vi "HexToDate.vi"(11 "数组":u16[](array[numeric]) format="%04xH") -> (3 "DATE":timestamp[](array[timestamp]))   [LabVIEW 2016, in "斯坦道总磷.lvlib"]
uses:
  <vilib>/Utility/miscctls.llb/LVDateTimeRec.ctl
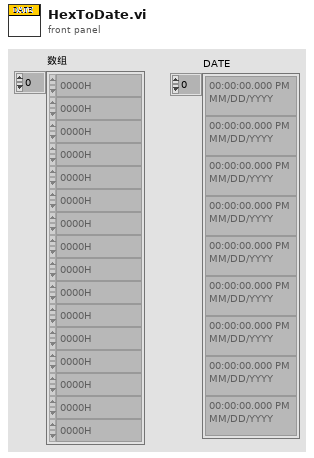
[diagram p1: front panel]
types:
  T1 = typedef "LVDateTimeRec.ctl" = cluster{"fractional second":dbl, "second":i32, "minute":i32, "hour":i32, "day of month":i32, "month":i32, "year":i32, "day of week":i32, "day of year":i32, "DST":i32}
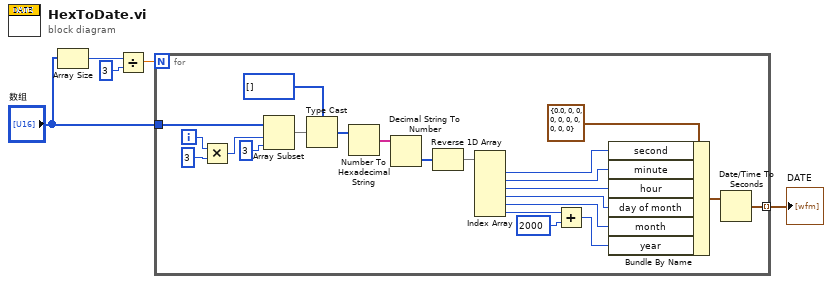
[diagram p0: block diagram]
diagram:
  n1 = Array Size(array="数组") -> (size(s)=w5:i32)
  n2 = Divide(x=w5, y=3) -> (x/y=w3:dbl)
  n3 = for {
    N: w3 -> [_]
    tunnel: "数组" -> [w27]
    tunnel: [w10] -> w1 mode=indexing
    i -> [w26]
    n4 = Multiply(x=w26, y=3) -> (x*y=w23:i32)
    n5 = Array Subset(array=w27, index=w23, length=3 ("索引")) -> (w22:u16[])
    n6 = Type Cast(type=u8[] [], x=w22) -> (*(type *) &x=w8:u8[])
    n7 = Number To Hexadecimal String(2:w8) -> (0:w7:string[])  [unwired: 1 in]
    n8 = Decimal String To Number(string=w7) -> (number=w6:i32[])  [unwired: 2 in, 1 out]
    n9 = Reverse 1D Array(array=w6) -> (reversed array=w9:i32[])
    n10 = Index Array(array=w9) -> (element #1=w19:i32, element #2=w18:i32, element #3=w17:i32, element #4=w16:i32, element #5=w15:i32, element #6=w14:i32)  [unwired: 6 in]
    n11 = Add(x=w14, y=2000) -> (x+y=w12:i32)
    n12 = Bundle By Name(cluster=T1 {"fractional second"=0.0, "second"=0, "minute"=0, "hour"=0, "day of month"=0, "month"=0, "year"=0, "day of week"=0, "day of year"=0, "DST"=0} ("日期时间记录"), "second"=w19, "minute"=w18, "hour"=w17, "day of month"=w16, "month"=w15, "year"=w12) -> (w11:T1)
    n13 = Date/Time To Seconds(2:w11) -> (0:w10:timestamp)  [unwired: 1 in]
  }
  "DATE" <- w1
